vi "Calculate_Height.vi"(9 "Z Value":dbl, 10 "Full top":cluster{"x":dbl, "y":dbl}[](array[cluster]), 11 "Base":cluster{"x":dbl, "y":dbl}[](array[cluster])) -> (3 "Adjusted top":cluster{"x":dbl, "y":dbl}[](array[cluster]))   [LabVIEW 2022 SP3]
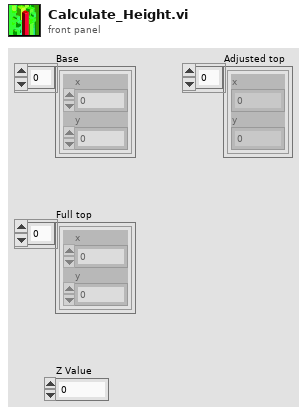
[diagram p1: front panel]
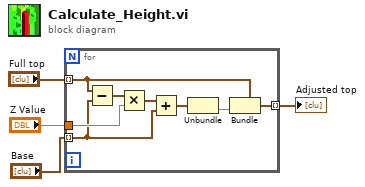
[diagram p0: block diagram]
diagram:
  n1 = for {
    tunnel: "Full top" -> [w9] mode=indexing
    tunnel: "Base" -> [w6] mode=indexing
    tunnel: "Z Value" -> [w11]
    tunnel: [w8] -> w4 mode=indexing
    n2 = Subtract(x=w9, y=w6) -> (x-y=w12:cluster{"x":dbl, "y":dbl})
    n3 = Multiply(x=w12, y=w11) -> (x*y=w7:cluster{"x":dbl, "y":dbl})
    n4 = Add(x=w7, y=w6) -> (x+y=w5:cluster{"x":dbl, "y":dbl})
    n5 = Unbundle(w5) -> ("y"=w10:dbl)  [unwired: 1 out]
    n6 = Bundle(cluster=w9, "y"=w10) -> (w8:cluster{"x":dbl, "y":dbl})  [unwired: 1 in]
  }
  "Adjusted top" <- w4
